vi "WFDC Messenger.vi"   [LabVIEW 2020]
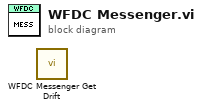
[diagram p0: block diagram]
diagram:
  n1 = call "WFDC Messenger Get Drift.vi"() -> ()  [unwired: 12 in, 4 out]
